vi "test_save_file.vi"() -> ()   [LabVIEW 2018]
panel:
  out "error out":errorcluster
  in  "stop":bool
  out "Graph":dbl[](graph)
  in  "File Path":string
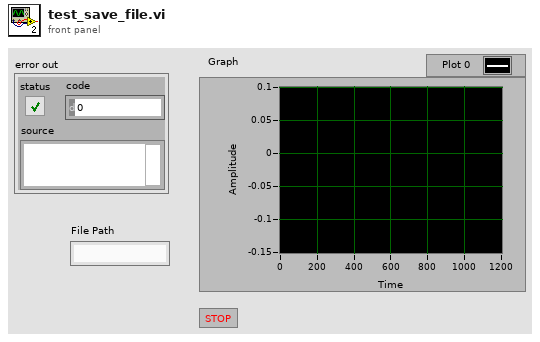
[diagram p1: front panel]
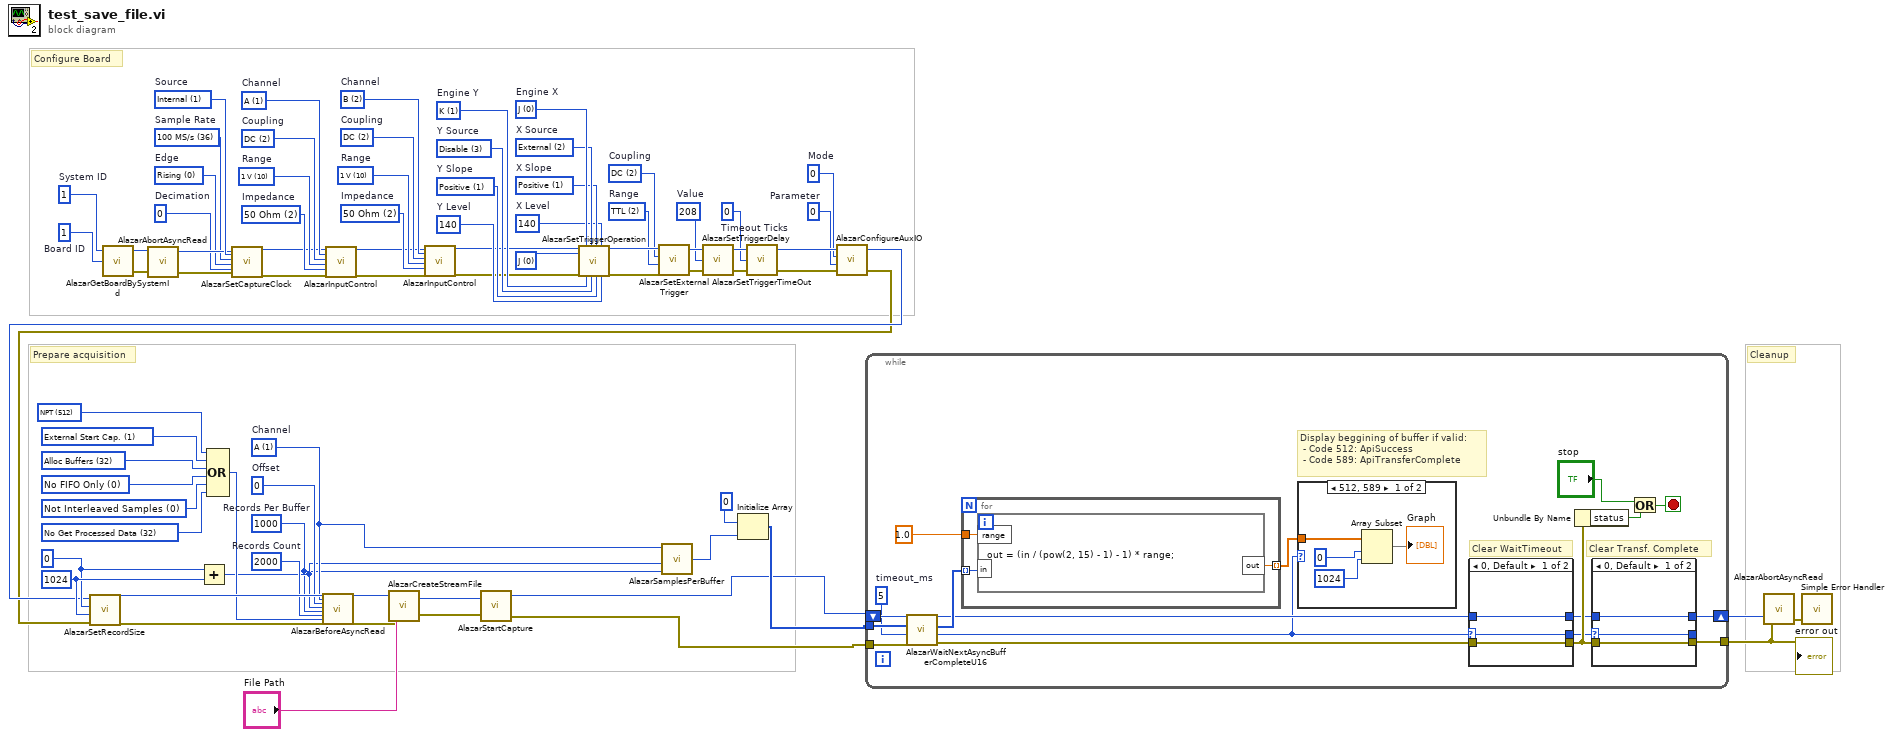
[diagram p0: block diagram]
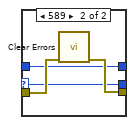
[diagram p3: hidden frame]
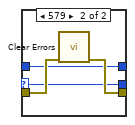
[diagram p4: hidden frame]
diagram:
  w46 = u32 2 items=["50 Ohm"=2]  # Impedance
  w45 = u32 10 items=["40 mV"=2, "100 mV"=5, "200 mV"=6, "400 mV"=7, "1 V"=10, "2 V"=11, "4 V"=12]  # Range
  w47 = u32 2 items=["AC"=1, "DC"=2]  # Coupling
  w48 = u8 2 items=["A"=1, "B"=2, "C"=4, "D"=8]  # Channel
  w24 = u32 0  # Parameter
  w23 = u32 0  # Mode
  w22 = u32 0  # Timeout Ticks
  w29 = u32 208  # Value
  w33 = u32 2 items=["5 V", "1 V", "TTL"]  # Range
  w32 = u32 2 items=["AC"=1, "DC"=2]  # Coupling
  w36 = u32 140  # Y Level
  w37 = u32 1 items=["Positive"=1, "Negative"=2]  # Y Slope
  w38 = u32 3 items=["A", "B", "External", "Disable", "C", "D"]  # Y Source
  w40 = u32 140  # X Level
  w41 = u32 1 items=["Positive"=1, "Negative"=2]  # X Slope
  w42 = u32 2 items=["A", "B", "External", "Disable", "C", "D"]  # X Source
  w39 = u32 1 items=["J", "K"]  # Engine Y
  w43 = u32 0 items=["J", "K"]  # Engine X
  w44 = u32 0 items=["J", "K", "J OR K", "J AND K", "J XOR K", "J AND NOT K", "NOT J AND K"] ("Op.")
  w51 = u32 2 items=["50 Ohm"=2]  # Impedance
  w52 = u32 10 items=["40 mV"=2, "100 mV"=5, "200 mV"=6, "400 mV"=7, "1 V"=10, "2 V"=11, "4 V"=12]  # Range
  w53 = u32 2 items=["AC"=1, "DC"=2]  # Coupling
  w54 = u8 1 items=["A"=1, "B"=2, "C"=4, "D"=8]  # Channel
  w56 = u32 0  # Decimation
  w57 = u32 0 items=["Rising", "Falling"]  # Edge
  w58 = u32 36 items=["1 kS/s"=1, "2 kS/s"=2, "5 kS/s"=4, "10 kS/s"=8, "20 kS/s"=10, "50 kS/s"=12, "100 kS/s"=14, "200 kS/s"=16, "500 kS/s"=18, "1 MS/s"=20, "2 MS/s"=24, "5 MS/s"=26, "10 MS/s"=28, "20 MS/s"=30, "50 MS/s"=34, "100 MS/s"=36, "125 MS/s"=37, "250 MS/s"=43, "500 MS/s"=48, "USER_DEF"=0]  # Sample Rate
  w60 = u32 1 items=["Internal"=1, "Fast External"=2, "Medium External"=3, "Slow External"=4, "External AC"=5, "External DC"=6, "External 10MHz"=7]  # Source
  w64 = u32 1  # Board ID
  w63 = u32 1  # System ID
  w66 = u32 2000  # Records Count
  w12 = u32 1000  # Records Per Buffer
  w67 = u32 0  # Offset
  w14 = u32 1 items=["A"=1, "B"=2, "A + B"=3, "C"=4, "A + C"=5, "A + B"=6, "D"=8, "A + D"=9, "B + D"=10, "C + D"=12, "A + B + C + D"=15]  # Channel
  w72 = u32 1024 ("Post-trigger Samples")
  w71 = u32 0 ("Pre-trigger Samples")
  w78 = u32 32 items=["No Get Processed Data"=32, "Get Processed Data"=8192]
  w77 = u32 0 items=["Not Interleaved Samples"=0, "Interleave Samples"=4096]
  w73 = u32 0 items=["No FIFO Only"=0, "FIFO Only"=2048]
  w76 = u32 32 items=["Alloc Buffers"=32]
  w75 = u32 1 items=["Internal Start Cap.", "External Start Cap."]
  w74 = u32 512 items=["Traditional"=0, "NPT"=512, "Continuous"=256, "Triggered Streaming"=1024]
  # "Cleanup"
  # "Configure Board"
  # "Prepare acquisition"
  n1 = call "AlazarGetBoardBySystemId.vi"("Board ID"=w64, "System ID"=w63) -> ("error out"=w61:errorcluster, "Handle"=w62:u32)  [unwired: 1 in, 1 out]
  n2 = call "AlazarAbortAsyncRead.vi"("Handle"=w62, "error in (no error)"=w61) -> ("Handle"=w59:u32, "error out"=w55:errorcluster)  [unwired: 1 out]
  n3 = Add(x=w71, y=w72) -> (x+y=w13:u32)
  n4 = Compound Arithmetic op=OR(w74, w75, w76, w73, w77, w78) -> (w68:u32)
  n5 = call "AlazarSetCaptureClock.vi"("Handle"=w59, "Source"=w60, "Sample Rate"=w58, "Edge"=w57, "Decimation"=w56, "error in (no error)"=w55) -> ("Handle"=w50:u32, "error out"=w49:errorcluster)  [unwired: 11 in, 1 out]
  n6 = call "AlazarInputControl.vi"("Handle"=w50, "Channel"=w54, "Coupling"=w53, "Range"=w52, "Impedance"=w51, "error in (no error)"=w49) -> ("Handle"=w21:u32, "error out"=w20:errorcluster)  [unwired: 11 in, 1 out]
  n7 = call "AlazarInputControl.vi"("Handle"=w21, "Channel"=w48, "Coupling"=w47, "Range"=w45, "Impedance"=w46, "error in (no error)"=w20) -> ("Handle"=w18:u32, "error out"=w19:errorcluster)  [unwired: 11 in, 1 out]
  n8 = call "AlazarSetTriggerOperation.vi"("Handle"=w18, "Trigger Operation"=w44, "error in (no error)"=w19, "Trigger Engine 1"=w43, "Trigger Engine 2"=w39, "Source 1"=w42, "Source 2"=w38, "Slope 1"=w41, "Slope 2"=w37, "Level 1"=w40, "Level 2"=w36) -> ("Handle"=w35:u32, "error out"=w34:errorcluster)  [unwired: 6 in, 1 out]
  n9 = call "AlazarSetExternalTrigger.vi"("error in (no error)"=w34, "Range ID"=w33, "Coupling ID"=w32, "Handle"=w35) -> ("error out"=w30:errorcluster, "Handle"=w31:u32)  [unwired: 1 out]
  n10 = call "AlazarSamplesPerBuffer.vi"("Records Per Buffer"=w12, "Samples Per Record"=w13, "Channel Mask"=w14) -> ("Samples Per Buffer"=w15:u32)  [unwired: 1 in]
  n11 = call "AlazarSetTriggerDelay.vi"("error in (no error)"=w30, "Delay"=w29, "Handle"=w31) -> ("error out"=w27:errorcluster, "Handle"=w28:u32)  [unwired: 1 out]
  n12 = Initialize Array(u16 0, w15) -> (w2:u16[])
  n13 = call "AlazarSetTriggerTimeOut.vi"("error in (no error)"=w27, "Timeout Ticks"=w22, "Handle"=w28) -> ("error out"=w25:errorcluster, "Handle"=w26:u32)  [unwired: 1 out]
  n14 = call "AlazarConfigureAuxIO.vi"("error in (no error)"=w25, "Parameter"=w24, "Mode"=w23, "Handle"=w26) -> ("error out"=w16:errorcluster, "Handle"=w17:u32)  [unwired: 1 out]
  n15 = call "AlazarSetRecordSize.vi"("error in (no error)"=w16, "Post-trigger Samples"=w72, "Pre-trigger Samples"=w71, "Handle"=w17) -> ("error out"=w69:errorcluster, "Handle"=w70:u32)  [unwired: 1 out]
  n16 = call "AlazarBeforeAsyncRead.vi"("Handle"=w70, "Channel Select"=w14, "Transfer Offset"=w67, "Transfer Length"=w13, "Records Per Buffer"=w12, "Records Per Acquisition"=w66, "Flags"=w68, "error in (no error)"=w69) -> ("Handle"=w11:u32, "error out"=w9:errorcluster)  [unwired: 17 in, 1 out]
  n17 = call "AlazarCreateStreamFile.vi"("error in (no error)"=w9, "File Path"="File Path", "Handle"=w11) -> ("error out"=w7:errorcluster, "Handle"=w8:u32)
  n18 = call "AlazarStartCapture.vi"("Handle"=w8, "error in (no error)"=w7) -> ("Handle"=w1:u32, "error out"=w3:errorcluster)  [unwired: 1 out]
  n19 = while {
    tunnel: w2 -> [w96]
    tunnel: w3 -> [w93]
    tunnel: [w85] -> w4
    shift-right: [w86] -> w5
    shift-left: w1 -> [w95]
    stop <- w89 stop-if-true
    w94 = u32 5  # timeout_ms
    # "Display beggining of buffer if valid:\n - Code 512: ApiSuccess\n - Code 589: ApiTransferComplete"
    # "Clear Transf. Complete"
    # "Clear WaitTimeout"
    n20 = call "AlazarWaitNextAsyncBufferCompleteU16.vi"("error in (no error)"=w93, "Timeout (ms)"=w94, "Buffer"=w96, "Handle"=w95) -> ("error out"=w81:errorcluster, "Return Code"=w79:u32, "Buffer"=w84:u16[], "Handle"=w82:u32)
    n21 = for {
      tunnel: w84 -> [w103] mode=indexing
      tunnel: sgl 1.0 -> [w102]
      tunnel: [w101] -> w80 mode=indexing
      n22 = formula code="out = (in / (pow(2, 15) - 1) - 1) * range;"("in"=w103, "range"=w102) -> ("out"=w101:dbl)
    }
    n23 = case shown="512, 589" w79 {
      tunnel: w80 -> [w97 _]
      frame 512, 589 {
        n24 = Array Subset(array=w97, index=0, length=1024) -> (→"Graph":dbl[])
      }
      frame Default {
      }
    }
    n25 = case shown="0, Default" w79 {
      selector: w79 -> [w112 w114]
      tunnel: w81 -> [w111 w117]
      tunnel: [w111 w116] -> w92
      tunnel: [w113 w115] -> w91
      tunnel: w82 -> [w113 w115]
      tunnel: [w112 w114] -> w90
      frame 0, Default {
      }
      frame 579 {
        n26 = call <vilib>:"Clear Errors.vi"("error in (no error)"=w117) -> ("error out"=w116:errorcluster)  [unwired: 5 in, 1 out]
      }
    }
    n27 = Unbundle By Name(w92) -> ("status"=w87:bool)
    n28 = case shown="0, Default" w90 {
      selector: w90 -> [w105 w107]
      tunnel: w92 -> [w104 w110]
      tunnel: [w104 w109] -> w85
      tunnel: [w106 w108] -> w86
      tunnel: w91 -> [w106 w108]
      tunnel: [w105 w107] -> _
      frame 0, Default {
      }
      frame 589 {
        n29 = call <vilib>:"Clear Errors.vi"("error in (no error)"=w110) -> ("error out"=w109:errorcluster)  [unwired: 5 in, 1 out]
      }
    }
    n30 = Or(x="stop", y=w87) -> (x .or. y?=w89:bool)
  }
  "error out" <- w4
  n31 = call "AlazarAbortAsyncRead.vi"("Handle"=w5, "error in (no error)"=w4) -> ("error out"=w6:errorcluster)  [unwired: 2 out]
  n32 = call <vilib>:"Simple Error Handler.vi"("error in (no error)"=w6) -> ()  [unwired: 4 in, 5 out]
